vi "Add Header.vi"(8 "error in":errorcluster, 9 "value":string, 10 "header":T1, 11 "session in":refnum<class "Session.lvclass">) -> (0 "error out":errorcluster, 3 "session out":refnum<class "Session.lvclass">)   [LabVIEW 2020, in "Library Commun.lvlib" / "Library Http.lvlib" / "Session.lvclass"]
doc: "Adds a header field line to future web requests associated with the HTTP session. Headers define attributes of the data exchanged between the client and server."
uses:
  Session.lvclass
  Header--Combo Box.ctl
  Session.lvclass/Session.ctl
  lvwebclient_32.dll
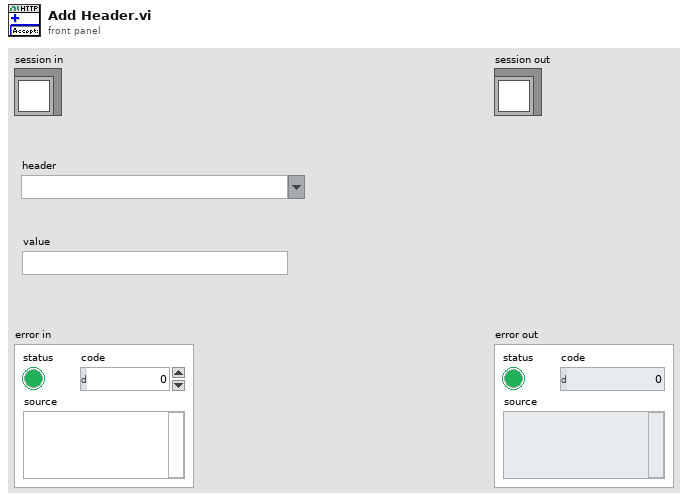
[diagram p1: front panel]
types:
  T1 = typedef "Library Commun.lvlib/Library Http.lvlib/Session.lvclass/Header--Combo Box.ctl" = string
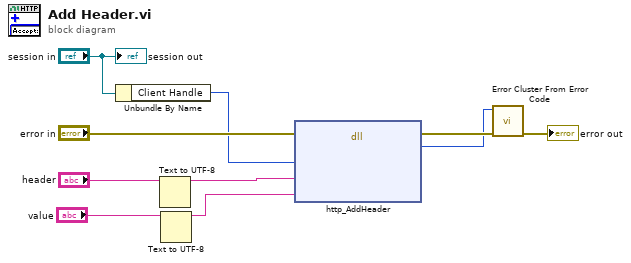
[diagram p0: block diagram]
diagram:
  n1 = Unbundle By Name("session in") -> ("Client Handle"=w5:u32)
  n2 = Text to UTF-8(11:"header") -> (3:w3:string)  [unwired: 2 in, 1 out]
  n3 = Text to UTF-8(11:"value") -> (3:w1:string)  [unwired: 2 in, 1 out]
  n4 = dll-call lib="C:/Users/ngarcin/OneDrive - Altyor/Standard TB/Class/Http Altyor/lvwebclient_*.*" fn="http_AddHeader"(error in="error in", "handle"=w5, "headerName"=w3, "headerValue"=w1) -> (error out=w7:errorcluster, "return"=w6:i32)  [unwired: 5 in, 1 out]
  n5 = call <vilib>:"Error Cluster From Error Code.vi"("error in (no error)"=w7, "error code (0)"=w6) -> ("error out"=→"error out":errorcluster)  [unwired: 7 in]
  "session out" <- "session in"
